vi "data_directory_create_if_nonexistant.vi"(2 "Cluster":T1, 3 "Tracker Handle":i32) -> (0 "Error":bool, 1 "Directory Exists?":bool)   [LabVIEW 2015]
uses:
  MWT.dll
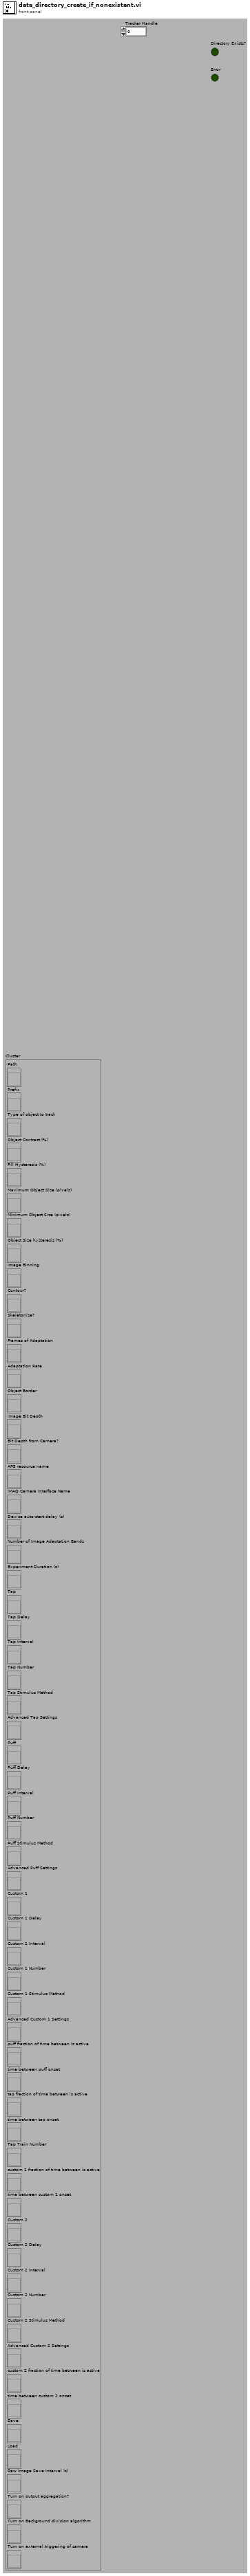
[diagram p1: front panel]
types:
  T1 = cluster{"Path":refnum<vi>, "Prefix":refnum<vi>, "Type of object to track":refnum<vi>, "Object Contrast (%)":refnum<vi>, "Fill Hysteresis (%)":refnum<vi>, "Maximum Object Size (pixels)":refnum<vi>, "Minimum Object Size (pixels)":refnum<vi>, "Object Size hysteresis (%)":refnum<vi>, "Image Binning":refnum<vi>, "Contour?":refnum<vi>, "Skeletonize?":refnum<vi>, "Frames of Adaptation":refnum<vi>, "Adaptation Rate":refnum<vi>, "Object Border":refnum<vi>, "Image Bit Depth":refnum<vi>, "Bit Depth from Camera?":refnum<vi>, "AFG resource name":refnum<vi>, "IMAQ Camera Interface Name":refnum<vi>, "Device auto-start delay (s)":refnum<vi>, "Number of Image Adaptation Bands":refnum<vi>, "Experiment Duration (s)":refnum<vi>, "Tap":refnum<vi>, "Tap Delay":refnum<vi>, "Tap Interval":refnum<vi>, "Tap Number":refnum<vi>, "Tap Stimulus Method":refnum<vi>, "Advanced Tap Settings":refnum<vi>, "Puff":refnum<vi>, "Puff Delay":refnum<vi>, "Puff Interval":refnum<vi>, "Puff Number":refnum<vi>, "Puff Stimulus Method":refnum<vi>, "Advanced Puff Settings":refnum<vi>, "Custom 1":refnum<vi>, "Custom 1 Delay":refnum<vi>, "Custom 1 Interval":refnum<vi>, "Custom 1 Number":refnum<vi>, "Custom 1 Stimulus Method":refnum<vi>, "Advanced Custom 1 Settings":refnum<vi>, "puff fraction of time between is active":refnum<vi>, "time between puff onset":refnum<vi>, "tap fraction of time between is active":refnum<vi>, "time between tap onset":refnum<vi>, "Tap Train Number":refnum<vi>, "custom 1 fraction of time between is active":refnum<vi>, "time between custom 1 onset":refnum<vi>, "Custom 2":refnum<vi>, "Custom 2 Delay":refnum<vi>, "Custom 2 Interval":refnum<vi>, "Custom 2 Number":refnum<vi>, "Custom 2 Stimulus Method":refnum<vi>, "Advanced Custom 2 Settings":refnum<vi>, "custom 2 fraction of time between is active":refnum<vi>, "time between custom 2 onset":refnum<vi>, "Save":refnum<vi>, "Load":refnum<vi>, "Raw Image Save Interval (s)":refnum<vi>, "Turn on output aggregation?":refnum<vi>, "Turn on Background division algorithm":refnum<vi>, "Turn on external triggering of camera":refnum<vi>}
  T2 = enum16{"open", "replace", "create", "open or create", "replace or create", "replace or create with confirmation"}
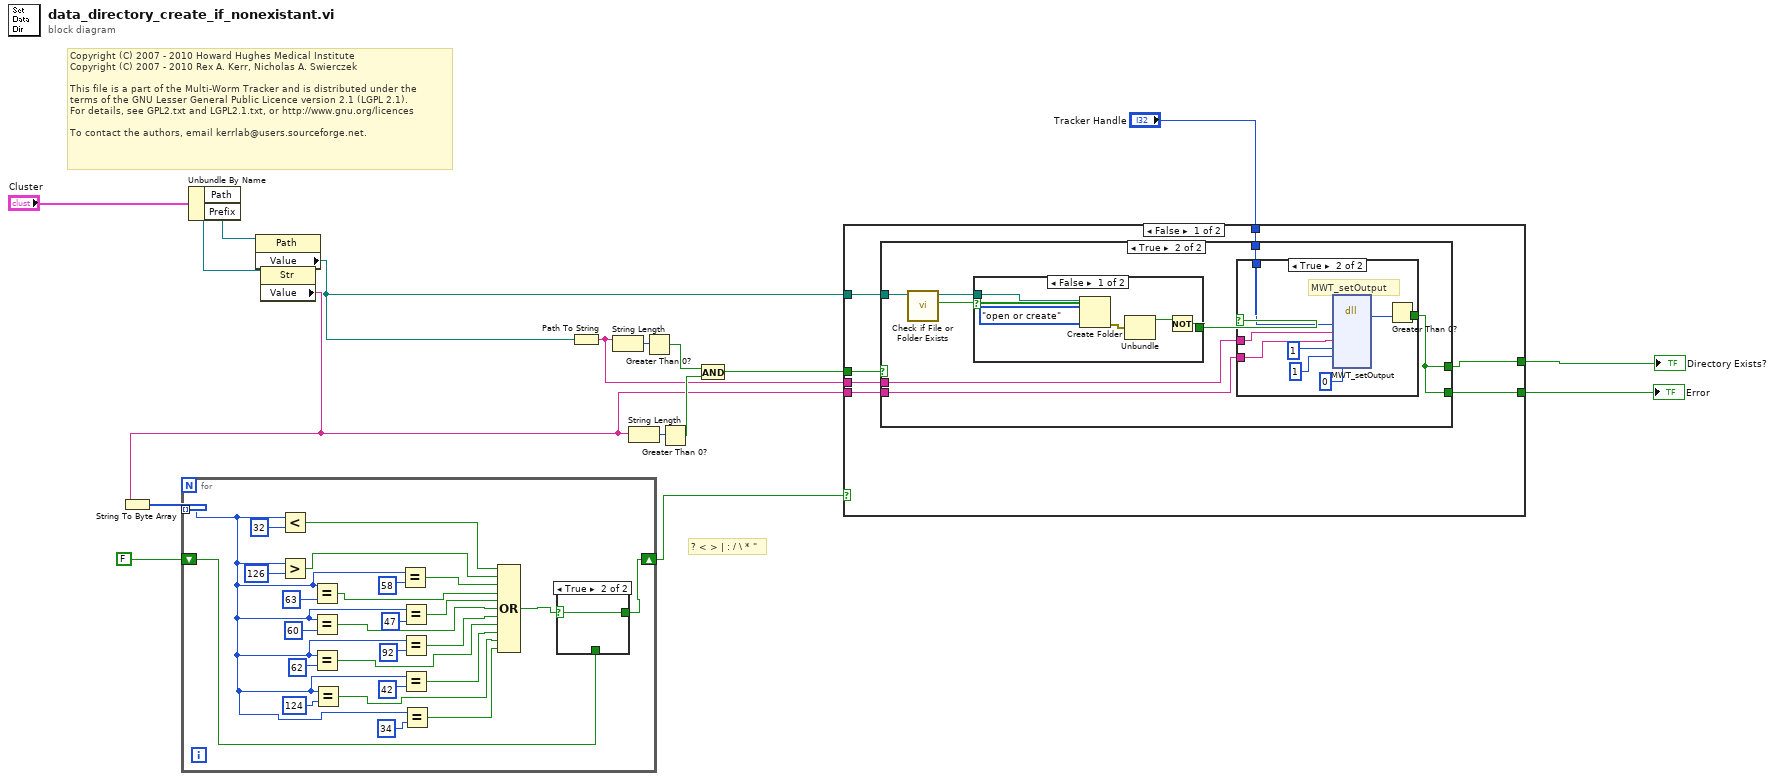
[diagram p0: block diagram]
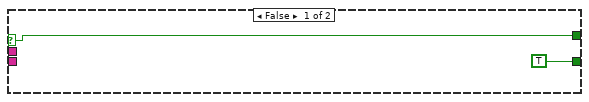
[diagram p2: hidden frame]
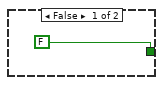
[diagram p3: hidden frame]
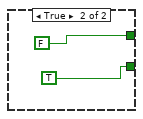
[diagram p5: hidden frame]
diagram:
  # "Copyright (C) 2007 - 2010 Howard Hughes Medical Institute\nCopyright (C) 2007 - 2010 Rex A. Kerr, Nicholas A. Swierczek\n \nThis file is a part of the Multi-Worm Tracker and is distributed under the\nterms of the GNU Lesser General Public Licence version 2.1 (LGPL 2.1).\nFor details, see GPL2.txt and LGPL2.1.txt, or http://www.gnu.org/licences\n \nTo contact the authors, email kerrlab@users.sourceforge.net."
  # "? < > | : / \\ * \""
  n1 = Unbundle By Name("Cluster") -> ("Path"=w10:refnum<vi>, "Prefix"=w9:refnum<vi>)
  n2 = property class="Path"(reference=w10) -> ("Value"=w8:path)  [unwired: 1 in, 2 out]
  n3 = property class="Str"(reference=w9) -> ("Value"=w5:string)  [unwired: 1 in, 2 out]
  n4 = String To Byte Array(string=w5) -> (unsigned byte array=w4:u8[])
  n5 = for {
    tunnel: w4 -> [w37] mode=indexing
    shift-right: [w19] -> w2
    shift-left: FALSE -> [w18]
    n6 = Less?(x=w37, y=u8 32) -> (x < y?=w31:bool)
    n7 = Greater?(x=w37, y=u8 126) -> (0:w30:bool)
    n8 = Equal?(x=w37, y=63) -> (x = y?=w28:bool)
    n9 = Equal?(x=w37, y=60) -> (x = y?=w26:bool)
    n10 = Equal?(x=w37, y=62) -> (x = y?=w24:bool)
    n11 = Equal?(x=w37, y=124) -> (x = y?=w22:bool)
    n12 = Equal?(x=w37, y=58) -> (x = y?=w29:bool)
    n13 = Equal?(x=w37, y=47) -> (x = y?=w27:bool)
    n14 = Equal?(x=w37, y=92) -> (x = y?=w25:bool)
    n15 = Equal?(x=w37, y=42) -> (x = y?=w23:bool)
    n16 = Equal?(x=w37, y=34) -> (x = y?=w21:bool)
    n17 = Compound Arithmetic op=OR(w31, w30, w29, w28, w27, w26, w25, w24, w23, w22, w21) -> (w20:bool)
    n18 = case shown="True" w20 {
      selector: w20 -> [_ w45]
      tunnel: [w44 w45] -> w19
      tunnel: w18 -> [w44 _]
      frame False {
      }
      frame True {
      }
    }
  }
  n19 = Path To String(path=w8) -> (string=w11:string)
  n20 = String Length(string=w11) -> (length=w16:i32)
  n21 = String Length(string=w5) -> (length=w13:i32)
  n22 = Greater Than 0?(x=w16) -> (x > 0?=w14:bool)
  n23 = Greater Than 0?(x=w13) -> (x > 0?=w12:bool)
  n24 = And(x=w14, y=w12) -> (x .and. y?=w15:bool)
  n25 = case shown="False" w2 {
    tunnel: [w52 FALSE] -> w17
    tunnel: w15 -> [w51 _]
    tunnel: w11 -> [w50 _]
    tunnel: w8 -> [w49 _]
    tunnel: "Tracker Handle" -> [w48 _]
    tunnel: [w47 TRUE] -> w6
    tunnel: w5 -> [w46 _]
    frame False {
      n26 = case shown="True" w51 {
        selector: w51 -> [w54 _]
        tunnel: [w54 w55] -> w52
        tunnel: w49 -> [_ w59]
        tunnel: w46 -> [_ w58]
        tunnel: w50 -> [_ w57]
        tunnel: w48 -> [_ w56]
        tunnel: [TRUE w55] -> w47
        frame False {
        }
        frame True {
          n27 = call <vilib>:"Check if File or Folder Exists.vi"("path"=w59) -> ("file or folder exists?"=w62:bool, "dup path"=w61:path)  [unwired: 8 in, 1 out]
          n28 = case shown="False" w62 {
            selector: w62 -> [_ w76]
            tunnel: w61 -> [w72 _]
            tunnel: [w73 w76] -> w60
            frame False {
              (unwired) T2."open or create" ("operation (0:open)")
              n29 = Create Folder(path (use dialog)=w72) -> (error out=w75:errorcluster)  [unwired: 2 in, 2 out]
              n30 = Unbundle(w75) -> ("status"=w74:bool)  [unwired: 2 out]
              n31 = Not(x=w74) -> (.not. x?=w73:bool)
            }
            frame True {
            }
          }
          n32 = case shown="True" w60 {
            tunnel: w58 -> [_ w70]
            tunnel: w57 -> [_ w71]
            tunnel: w56 -> [_ w69]
            tunnel: [FALSE w67] -> w55
            frame False {
            }
            frame True {
              # "MWT_setOutput"
              n33 = dll-call lib="C:/Users/ramasamyl/Desktop/MWT/MWT.dll" fn="MWT_setOutput"("handle"=w69, "path"=w71, "prefix"=w70, "save_obj"=1, "save_ref"=1, "save_im"=0 ("save_obj")) -> ("return type"=w68:i32)  [unwired: 9 in, 2 out]
              n34 = Greater Than 0?(x=w68) -> (x > 0?=w67:bool)
            }
          }
        }
      }
    }
    frame True {
    }
  }
  "Directory Exists?" <- w17
  "Error" <- w6
